vi "Stop Lockin Sweep.vi"(8 "error in (no error)":errorcluster, 11 "MeasurementSMO in":refnum<class "MeasurementSMO.lvclass">) -> (0 "error out":errorcluster, 3 "MeasurementSMO out":refnum<class "MeasurementSMO.lvclass">)   [LabVIEW 2019, in "MeasurementSMO.lvclass"]
uses:
  MeasurementSMO.lvclass
  ab76b46b-8641-4e99-8c09-0fc40caff8b8.vi
  <userlib>/LevyLab/Lockin-Multichannel/Instrument.Lockin/Instrument.Lockin.lvclass
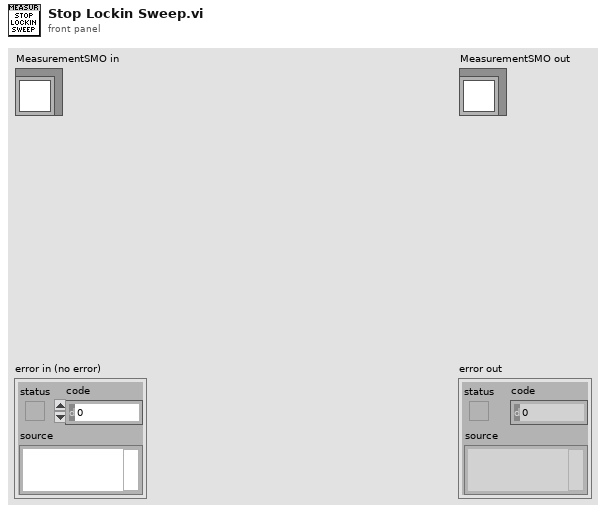
[diagram p1: front panel]
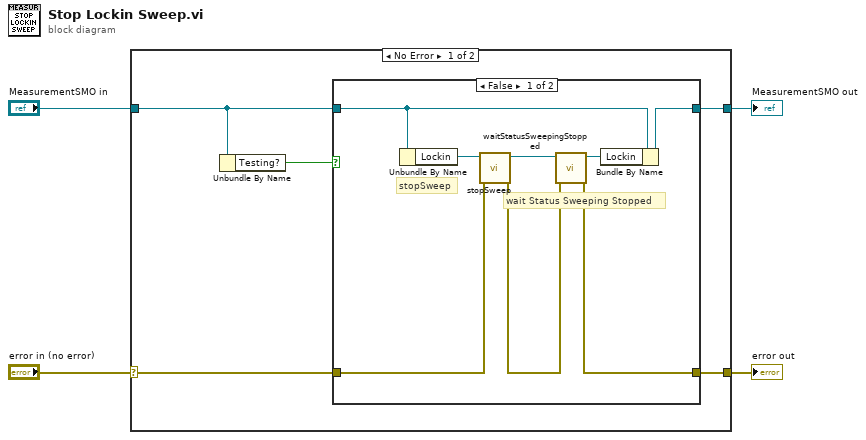
[diagram p0: block diagram]
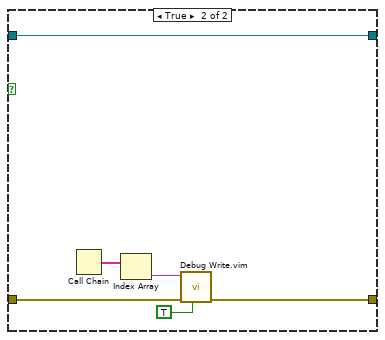
[diagram p2: hidden frame]
diagram:
  n1 = case shown="No Error" "error in (no error)" {
    selector: "error in (no error)" -> [w8 w25]
    tunnel: [w9 w25] -> w3
    tunnel: [w7 w24] -> w1
    tunnel: "MeasurementSMO in" -> [w5 w24]
    frame No Error {
      n2 = Unbundle By Name(w5) -> ("Testing?"=w6:bool)
      n3 = case shown="False" w6 {
        tunnel: [w10 w20] -> w9
        tunnel: w8 -> [w14 w19]
        tunnel: [w17 w23] -> w7
        tunnel: w5 -> [w16 w23]
        frame False {
          # "wait Status Sweeping Stopped"
          # "stopSweep"
          n4 = Unbundle By Name(w16) -> ("Lockin"=w15:refnum<class "Instrument.Lockin.lvclass">)
          n5 = call <userlib>:"stopSweep.vi"("error in (no error)"=w14, "Instrument.Lockin in"=w15) -> ("error out"=w11:errorcluster, "Instrument.Lockin out"=w13:refnum<class "Instrument.Lockin.lvclass">)  [unwired: 8 in]
          n6 = call <userlib>:"waitStatusSweepingStopped.vi"("error in (no error)"=w11, "Instrument.Lockin in"=w13) -> ("error out"=w10:errorcluster, "Instrument.Lockin out"=w12:refnum<class "Instrument.Lockin.lvclass">)  [unwired: 8 in]
          n7 = Bundle By Name(cluster=w16, "Lockin"=w12) -> (w17:refnum<class "MeasurementSMO.lvclass">)
        }
        frame True {
          n8 = Call Chain() -> (call chain=w22:string[])
          n9 = Index Array(array=w22) -> (element=w21:string)  [unwired: 1 in]
          n10 = call "Debug Write.vim"("include timestamp? (F)"=TRUE, "error in (no error)"=w19, "value"=w21) -> ("error out"=w20:errorcluster)  [unwired: 8 in]
        }
      }
    }
    frame Error {
    }
  }
  "error out" <- w3
  "MeasurementSMO out" <- w1
